vi "Ke2000 Auto Range.vi"(8 "error in (no error)":errorcluster, 10 "AUTO ON/OFF":bool, 11 "VISA resource name":refnum<visa-resource-name>) -> (0 "error out":errorcluster, 3 "VISA resource name out":refnum<visa-resource-name>)   [LabVIEW 2012]
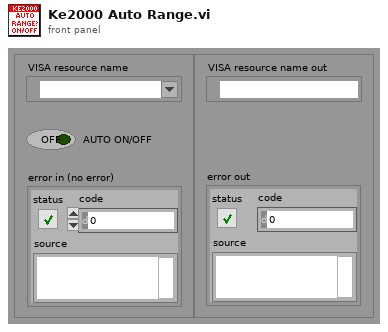
[diagram p1: front panel]
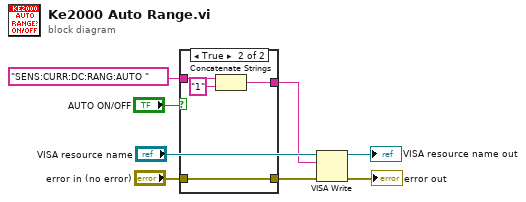
[diagram p0: block diagram]
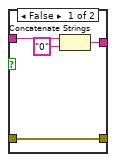
[diagram p2: hidden frame]
diagram:
  n1 = case shown="True" "AUTO ON/OFF" {
    tunnel: "SENS:CURR:DC:RANG:AUTO " ("write buffer") -> [w11 w16]
    tunnel: [w12 w14] -> w4
    tunnel: "error in (no error)" -> [w9 w13]
    tunnel: [w9 w13] -> w1
    frame False {
      n2 = Concatenate Strings(w11, "0" ("string")) -> (w12:string)
    }
    frame True {
      n3 = Concatenate Strings(w16, "1" ("string")) -> (w14:string)
    }
  }
  n4 = VISA Write(VISA resource name="VISA resource name", write buffer=w4, error in (no error)=w1) -> (VISA resource name out=→"VISA resource name out":refnum<visa-resource-name>, error out=→"error out":errorcluster)  [unwired: 1 out]
